vi "PostError.vi"(8 "error in (no error)":errorcluster, 9 "Type":T1, 10 "Message":string, 11 "ErrorManager in":refnum<class "ErrorManager.lvclass">) -> (0 "error out":errorcluster, 3 "ErrorManager out":refnum<class "ErrorManager.lvclass">)   [LabVIEW 2020, in "ErrorManager.lvlib" / "ErrorManager.lvclass"]
uses:
  ErrorManager.lvclass
  obj/Addons/LabVIEWObjectInterfaces.lvlibp/ErrorManager/ErrorManager/ErrorType.ctl
  ErrorInfo.ctl
  ErrorManager.lvclass/ErrorManager.ctl
  obj/Addons/LabVIEWObjectInterfaces.lvlibp/LabVIEWObjectInterfaces/IErrorManager/IErrorManager.lvclass
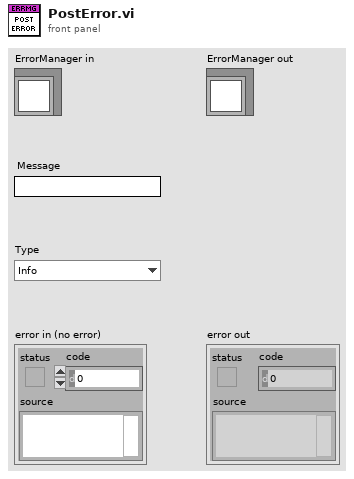
[diagram p1: front panel]
types:
  T1 = typedef "LabVIEWObjectInterfaces.lvlibp/IErrorManager.lvclass/ErrorType.ctl" = enum16{"Info", "Warning", "Error"}
  T2 = typedef "ErrorManager.lvlib/ErrorManager.lvclass/ErrorInfo.ctl" = cluster{"Time Stamp":timestamp, "Message":string, "Type":T1}
  T3 = typedef "ErrorManager.lvlib/ErrorManager.lvclass/ErrorInfoArrayRef.ctl" = refnum<data-value>
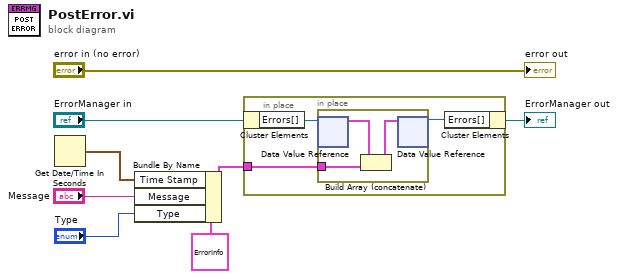
[diagram p0: block diagram]
diagram:
  n1 = Get Date/Time In Seconds() -> (seconds since 1Jan1904=w4:timestamp)
  n2 = Bundle By Name(cluster=T2 {"Time Stamp"=timestamp(0 s since 1904-01-01), "Message"="", "Type"=enum."Info"} ("Error Info"), "Time Stamp"=w4, "Message"="Message", "Type"="Type") -> (w2:T2)
  n3 = in-place {
    in-place-border: w2 -> [w9]
    n4 = in-place-cluster #1("ErrorManager in") -> ("Errors[]"=w11:T3)
    n5 = in-place {
      in-place-border: w9 -> [w13]
      n6 = in-place-dvr #2(w11) -> (w14:T2[])  [unwired: 1 out]
      n7 = Build Array (concatenate)(w14, w13) -> (w12:T2[])
      n8 = in-place-dvr #2(w12) -> (w10:T3)  [unwired: 1 out]
    }
    n9 = in-place-cluster #1("Errors[]"=w10) -> (→"ErrorManager out":refnum<class "ErrorManager.lvclass">)
  }
  "error out" <- "error in (no error)"
